vi "mainFIFO_2.vi"() -> ()   [LabVIEW 2018]
uses:
  <vilib>/rvi/Emulation/niFpgaGetClockAttributes.vi
  <vilib>/rvi/Emulation/niFpgaSctlEmulationGetInTimedLoop.vi
  <vilib>/rvi/Emulation/niFpgaEmulationReportErrorSimple.vi
  <vilib>/rvi/eio/common/nirviEmuTemplateMethod_errors.vi
  <vilib>/rvi/interface/RandomDataEmulation/niFpgaRandomDataHandleErrors.vi
  <vilib>/rvi/Emulation/niFpgaCriticalErrorInLSC.vi
  <vilib>/eio/EIONode/EIONode.xnode
  <vilib>/rvi/DataTransferAndStorage/Container/XNode/niFpgaContainer.xnode
  <vilib>/rvi/interface/RandomDataEmulation/nirviRandomDataFpgaReadWriteTemplate.vi
panel:
  out "data":u16[](array[numeric])
  out "dataFifoFull":bool
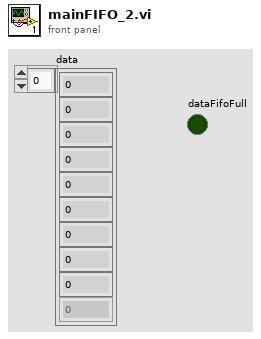
[diagram p1: front panel]
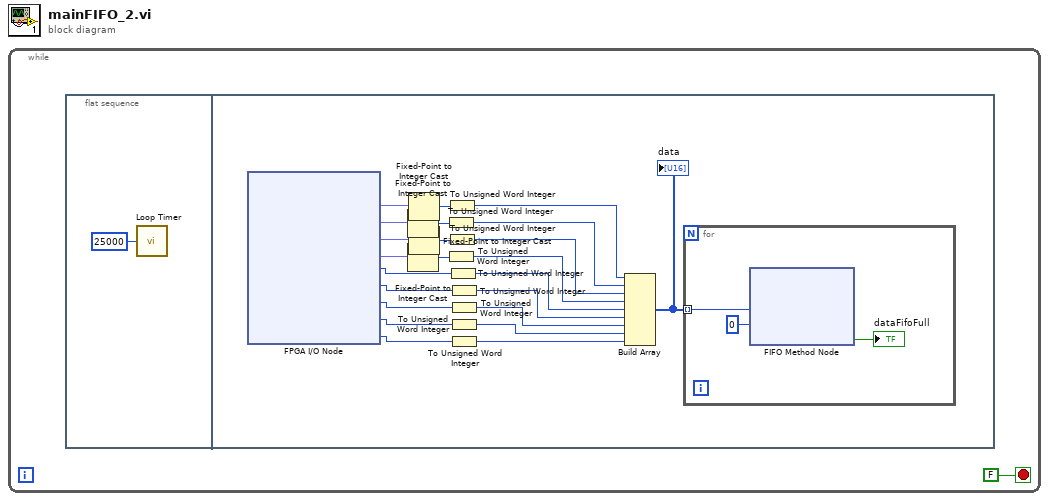
[diagram p0: block diagram]
diagram:
  n1 = while {
    stop <- FALSE stop-if-true
    n2 = flat-sequence {
      frame #0 {
        n3 = call "Loop Timer"("Count(uSec)"=u32 25000) -> ()  [unwired: 1 out]
      }
      frame #1 {
        n4 = xnode "FPGA I/O Node"() -> ("ilcMotorCurrent"=w14:fxp<+/-,16,5>, "ilcCommCurrent"=w10:fxp<+/-,16,5>, "ilcMotorVoltage"=w7:fxp<+/-,16,7>, "ilcCommVoltage"=w6:fxp<+/-,16,7>, "Mod4/CH7:0"=w25:u8, "Mod5/DI7:0"=w24:u8, "Mod5/DI15:8"=w23:u8, "Mod5/DI23:16"=w22:u8, "Mod5/DI31:24"=w21:u8)  [unwired: 9 in, 9 out]
        n5 = Fixed-Point to Integer Cast(1:w10) -> (0:w11:i16)
        n6 = Fixed-Point to Integer Cast(1:w6) -> (0:w9:i16)
        n7 = Fixed-Point to Integer Cast(1:w14) -> (0:w13:i16)
        n8 = Fixed-Point to Integer Cast(1:w7) -> (0:w8:i16)
        n9 = To Unsigned Word Integer(number=w11) -> (unsigned 16bit integer=w5:u16)
        n10 = To Unsigned Word Integer(number=w9) -> (unsigned 16bit integer=w3:u16)
        n11 = To Unsigned Word Integer(number=w13) -> (unsigned 16bit integer=w12:u16)
        n12 = To Unsigned Word Integer(number=w8) -> (unsigned 16bit integer=w4:u16)
        n13 = To Unsigned Word Integer(number=w25) -> (unsigned 16bit integer=w20:u16)
        n14 = To Unsigned Word Integer(number=w24) -> (unsigned 16bit integer=w19:u16)
        n15 = To Unsigned Word Integer(number=w23) -> (unsigned 16bit integer=w18:u16)
        n16 = To Unsigned Word Integer(number=w22) -> (unsigned 16bit integer=w17:u16)
        n17 = To Unsigned Word Integer(number=w21) -> (unsigned 16bit integer=w16:u16)
        n18 = Build Array(w12, w5, w4, w3, w20, w19, w18, w17, w16) -> (w15:u16[])
        "data" <- w15
        n19 = for {
          tunnel: w15 -> [w27] mode=indexing
          n20 = xnode ("FIFO Method Node")("Element"=w27, "Timeout"=0) -> ("Timed Out?"=→"dataFifoFull":bool)  [unwired: 1 in, 1 out]
        }
      }
    }
  }
